vi "Insert Result Data.vi"(8 "error in (no error)":errorcluster, 10 "GRR Results":T1[](array[typedef]), 11 "Session Handle in":T2) -> (0 "error out":errorcluster, 3 "Session Handle out":T2)   [LabVIEW 2018, in "Result Data Mgr.lvclass"]
uses:
  Result Data Mgr.lvclass
  Typedefs/Session Handle.ctl
  Typedefs/GRR Result.ctl
  Result Data Mgr.lvclass/Result Data Mgr.ctl
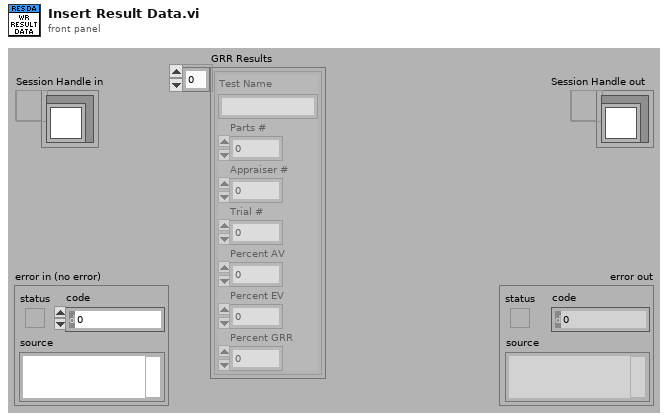
[diagram p1: front panel]
types:
  T1 = typedef "Result Data Mgr.lvclass/GRR Result.ctl" = cluster{"Test Name":string, "Parts #":u8, "Appraiser #":u8, "Trial #":u8, "Percent AV":dbl, "Percent EV":dbl, "Percent GRR":dbl}
  T2 = typedef "Result Data Mgr.lvclass/Session Handle.ctl" = refnum<data-value>
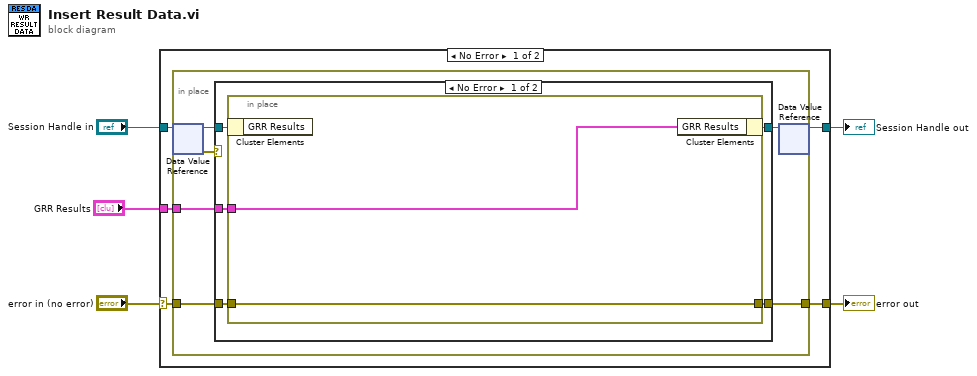
[diagram p0: block diagram]
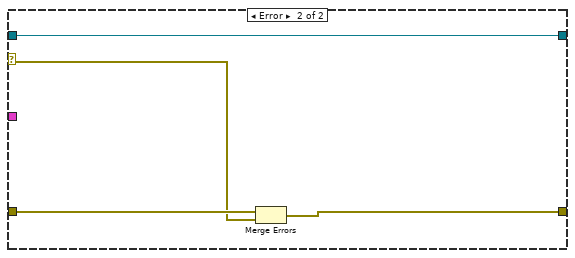
[diagram p2: hidden frame]
diagram:
  n1 = case shown="No Error" "error in (no error)" {
    selector: "error in (no error)" -> [w8 w28]
    tunnel: "Session Handle in" -> [w10 w29]
    tunnel: [w9 w29] -> w4
    tunnel: [w7 w28] -> w3
    tunnel: "GRR Results" -> [w6 _]
    frame No Error {
      n2 = in-place {
        in-place-border: w8 -> [w12]
        in-place-border: [w15] -> w7
        in-place-border: w6 -> [w11]
        n3 = in-place-dvr #1(w10) -> (w16:refnum<class "Result Data Mgr.lvclass">, w13:errorcluster)
        n4 = case shown="No Error" w13 {
          selector: w13 -> [_ w26]
          tunnel: w16 -> [w21 w24]
          tunnel: [w20 w25] -> w15
          tunnel: [w19 w24] -> w14
          tunnel: w12 -> [w18 w27]
          tunnel: w11 -> [w17 _]
          frame No Error {
            n5 = in-place {
              in-place-border: [w23] -> w20
              in-place-border: w18 -> [w23]
              in-place-border: w17 -> [w22]
              n6 = in-place-cluster #2(w21) -> ()  [unwired: 1 out]
              n7 = in-place-cluster #2("GRR Results"=w22) -> (w19:refnum<class "Result Data Mgr.lvclass">)
            }
          }
          frame Error {
            n8 = Merge Errors(w27, w26) -> (w25:errorcluster)
          }
        }
        n9 = in-place-dvr #1(w14) -> (w9:T2)  [unwired: 1 out]
      }
    }
    frame Error {
    }
  }
  "Session Handle out" <- w4
  "error out" <- w3
